vi "Test Karty (RS232).vi"() -> ()   [LabVIEW 2014]
uses:
  Kontrolki/KartaDAQ/CONF AI HW config.ctl
  <vilib>/Instr/_visa.llb/VISA Configure Serial Port (Instr).vi
panel:
  out "write buffer 2":string
  in  "VISA resource name":refnum<visa-resource-name>="COM3"
  in  "Przeslij ponwnie":bool
  out "AI HW config":T1
  in  "Zakres":enum16{"1000V", "300V", "30V", "3V", "0,3V"}(ring)
  out "error out":errorcluster
  in  "stop":bool
  out "read buffer":string
  out "write buffer":string
  # "LSB"
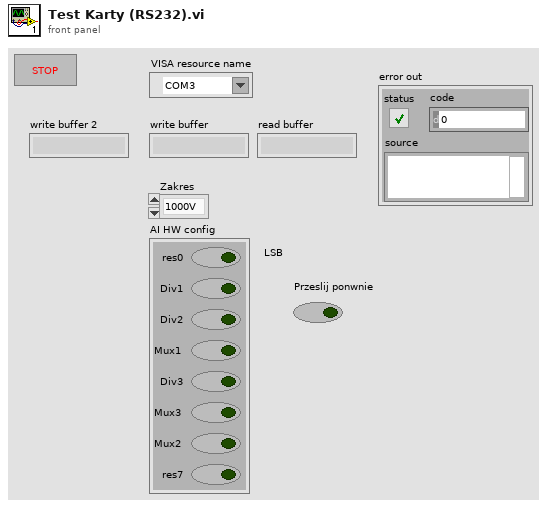
[diagram p1: front panel]
types:
  T1 = typedef "CONF AI HW config.ctl" = cluster{"res0":bool, "Div1":bool, "Div2":bool, "Mux1":bool, "Div3":bool, "Mux3":bool, "Mux2":bool, "res7":bool}
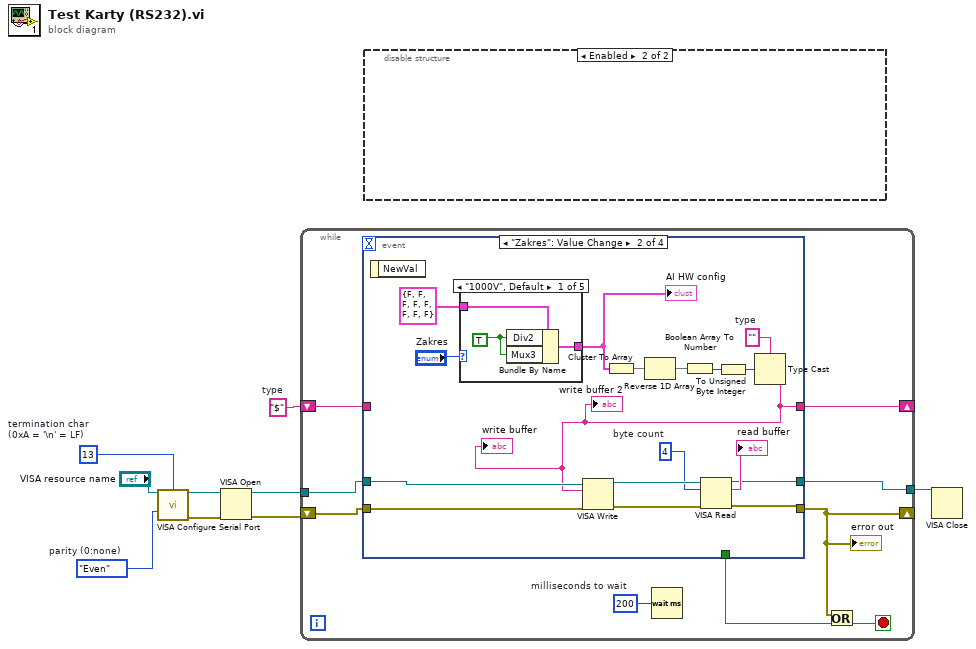
[diagram p0: block diagram]
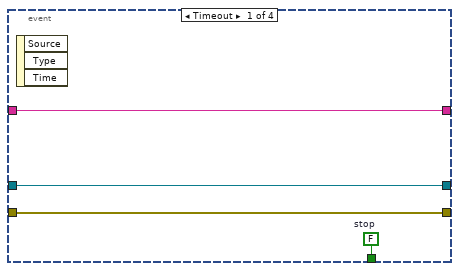
[diagram p3: hidden frame]
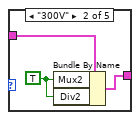
[diagram p4: hidden frame]
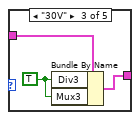
[diagram p5: hidden frame]
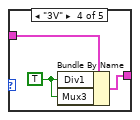
[diagram p6: hidden frame]
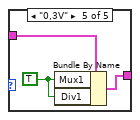
[diagram p7: hidden frame]
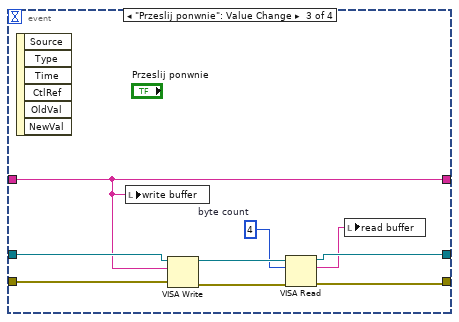
[diagram p8: hidden frame]
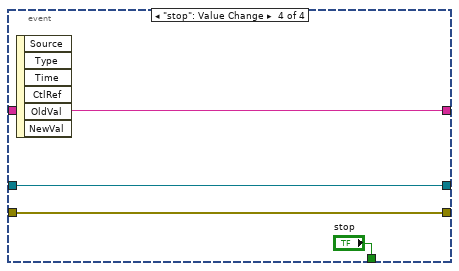
[diagram p9: hidden frame]
diagram:
  w1 = "$"  # type
  w2 = u8 13  # termination char (0xA = '\n' = LF)
  w3 = enum16{"None", "Odd", "Even", "Mark", "Space"}."Even"  # parity (0:none)
  n1 = call-poly "VISA Configure Serial Port"("VISA resource name"="VISA resource name", "termination char\n(0xA = '\\n' = LF)"=w2, "parity (0:none)"=w3) -> ("VISA resource name out"=w8:refnum<visa-resource-name>, "error out"=w9:errorcluster)  [unwired: 11 in]
  n2 = VISA Open(error in (no error)=w9, VISA resource name=w8) -> (VISA resource name=w6:refnum<visa-resource-name>, error out=w7:errorcluster)  [unwired: 3 in]
  n3 = while {
    tunnel: w6 -> [w16]
    tunnel: [w13] -> w5
    shift-right: [w14] -> _
    shift-left: w7 -> [w15]
    shift-right: [w10] -> _
    shift-left: w1 -> [w11]
    stop <- w18 stop-if-true
    w17 = u32 200  # milliseconds to wait
    n4 = event shown="[1] \"Zakres\": Value Change" {
      selector: _ -> [_ _ _ _]
      dyn-events: _ -> [_ _ _ _]
      timeout: _ -> [_ _ _ _]
      tunnel: w16 -> [w21 w31 w60 w67]
      tunnel: w15 -> [w22 w30 w59 w66]
      tunnel: [w22 w28 w58 w66] -> w14
      tunnel: [w21 w29 w57 w67] -> w13
      tunnel: [w20 _ _ "stop"] -> w12
      tunnel: w11 -> [w19 _ w55 w64]
      tunnel: [w19 w23 w55 w64] -> w10
      event Timeout {
        w20 = FALSE  # stop
        n5 = event-data() -> ()  [unwired: 1 in, 3 out]
      }
      event "Zakres": Value Change {
        w33 = u32 4  # byte count
        w36 = ""  # type
        n6 = event-data() -> ()  [unwired: 1 in, 1 out]
        n7 = case shown="\"1000V\", Default" "Zakres" {
          tunnel: T1 {"res0"=FALSE, "Div1"=FALSE, "Div2"=FALSE, "Mux1"=FALSE, "Div3"=FALSE, "Mux3"=FALSE, "Mux2"=FALSE, "res7"=FALSE} ("AI HW config") -> [w42 w45 w48 w51 w54]
          tunnel: [w41 w44 w47 w50 w53] -> w37
          frame "1000V", Default {
            w40 = TRUE ("Mux1")
            n8 = Bundle By Name(cluster=w42, "Div2"=w40, "Mux3"=w40) -> (w41:T1)
          }
          frame "300V" {
            w43 = TRUE ("Mux1")
            n9 = Bundle By Name(cluster=w45, "Mux2"=w43, "Div2"=w43) -> (w44:T1)
          }
          frame "30V" {
            w46 = TRUE ("Mux1")
            n10 = Bundle By Name(cluster=w48, "Div3"=w46, "Mux3"=w46) -> (w47:T1)
          }
          frame "3V" {
            w49 = TRUE ("Mux1")
            n11 = Bundle By Name(cluster=w51, "Div1"=w49, "Mux3"=w49) -> (w50:T1)
          }
          frame "0,3V" {
            w52 = TRUE ("Mux1")
            n12 = Bundle By Name(cluster=w54, "Mux1"=w52, "Div1"=w52) -> (w53:T1)
          }
        }
        "AI HW config" <- w37
        n13 = Cluster To Array(cluster=w37) -> (array=w25:bool[])
        n14 = Reverse 1D Array(array=w25) -> (reversed array=w24:bool[])
        n15 = Boolean Array To Number(Boolean array=w24) -> (number=w26:u32)
        n16 = To Unsigned Byte Integer(number=w26) -> (unsigned 8bit integer=w27:u8)
        n17 = Type Cast(type=w36, x=w27) -> (*(type *) &x=w23:string)
        "write buffer" <- w23
        "write buffer 2" <- w23
        n18 = VISA Write(VISA resource name=w31, write buffer=w23, error in (no error)=w30) -> (VISA resource name out=w34:refnum<visa-resource-name>, error out=w35:errorcluster)  [unwired: 1 out]
        n19 = VISA Read(VISA resource name=w34, byte count=w33, error in (no error)=w35) -> (VISA resource name out=w29:refnum<visa-resource-name>, read buffer=→"read buffer":string, error out=w28:errorcluster)  [unwired: 1 out]
      }
      event "Przeslij ponwnie": Value Change {
        w61 = u32 4  # byte count
        n20 = event-data() -> ()  [unwired: 1 in, 6 out]
        n21 = local write "write buffer"(w55) -> ()
        n22 = VISA Write(VISA resource name=w60, write buffer=w55, error in (no error)=w59) -> (VISA resource name out=w62:refnum<visa-resource-name>, error out=w63:errorcluster)  [unwired: 1 out]
        n23 = VISA Read(VISA resource name=w62, byte count=w61, error in (no error)=w63) -> (VISA resource name out=w57:refnum<visa-resource-name>, read buffer=w56:string, error out=w58:errorcluster)  [unwired: 1 out]
        n24 = local write "read buffer"(w56) -> ()
      }
      event "stop": Value Change {
        n25 = event-data() -> ()  [unwired: 1 in, 6 out]
      }
    }
    "error out" <- w14
    n26 = Wait (ms)(milliseconds to wait=w17) -> ()  [unwired: 1 out]
    n27 = Or(x=w14, y=w12) -> (x .or. y?=w18:bool)
  }
  n28 = disable-structure shown="Enabled" {
    frame Disabled {
    }
    frame Enabled {
    }
  }
  n29 = VISA Close(VISA resource name=w5) -> ()  [unwired: 1 in, 1 out]
